vi "Separate_Bits.vi"(0 "JSON":string, 7 "int size number":u32, 11 "error in":errorcluster) -> (4 "Value_string":string, 8 "hex_data":string, 15 "error out":errorcluster)   [LabVIEW 2021]
uses:
  <vilib>/JDP Science/JSONtext/String Subset.vi
  <vilib>/JDP Science/JSONtext/support/Strip Quotes and Unescape.vi
  <vilib>/JDP Science/JSONtext/support/Unescape JSON string.vi
  <vilib>/JDP Science/JSONtext/Parsing/Parse Full Path or Item Name.vi
  <vilib>/JDP Science/JSONtext/Offset/Find Item Locations by Path.vi
  <vilib>/JDP Science/JSONtext/JSONtext.lvlib
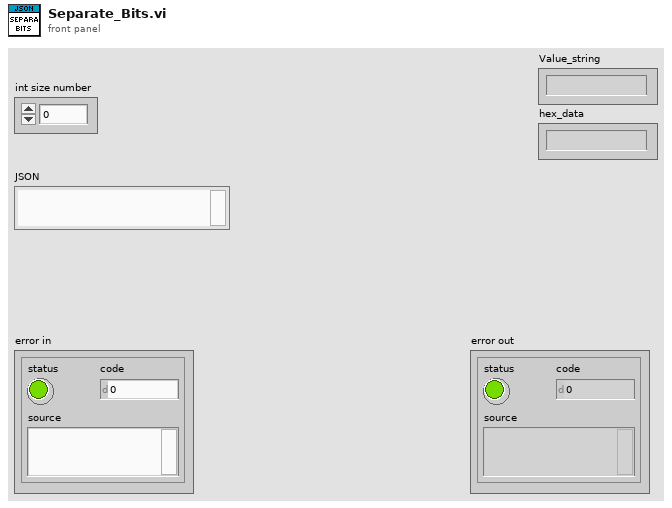
[diagram p1: front panel]
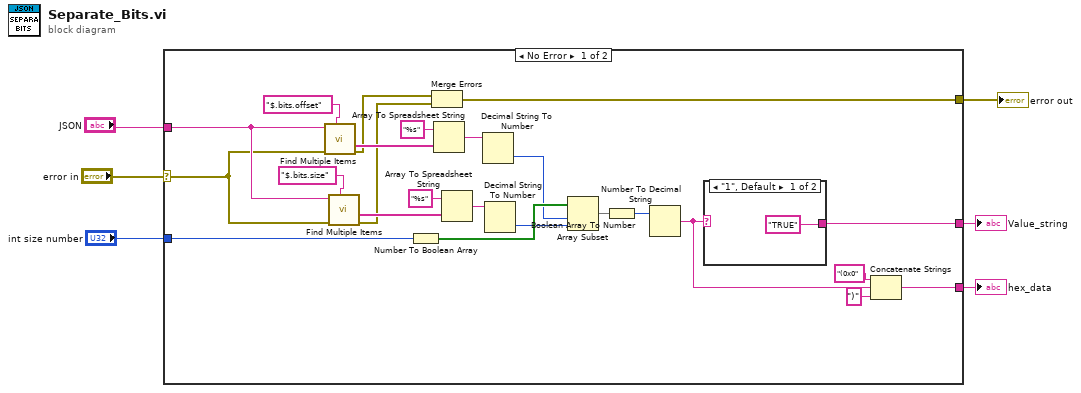
[diagram p0: block diagram]
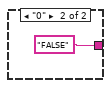
[diagram p2: hidden frame]
diagram:
  n1 = case shown="No Error" "error in" {
    selector: "error in" -> [w13 w33]
    tunnel: "int size number" -> [w15 _]
    tunnel: "JSON" -> [w14 _]
    tunnel: [w12 _] -> w2
    tunnel: [w11 _] -> w1
    tunnel: [w8 w33] -> w3
    frame No Error {
      n2 = call <vilib>:"Find Multiple Items.vi"("$Path or Item Name"="$.bits.offset", "error in (no error)"=w13, "JSON"=w14) -> ("error out"=w10:errorcluster, "<JSON>"=w19:string[])  [unwired: 5 in, 2 out]
      n3 = call <vilib>:"Find Multiple Items.vi"("$Path or Item Name"="$.bits.size", "error in (no error)"=w13, "JSON"=w14) -> ("error out"=w9:errorcluster, "<JSON>"=w24:string[])  [unwired: 5 in, 2 out]
      n4 = Number To Boolean Array(number=w15) -> (Boolean array=w28:bool[])
      n5 = Merge Errors(w10, w9) -> (w8:errorcluster)
      n6 = Array To Spreadsheet String(array=w19, 3:"%s" ("format string")) -> (spreadsheet string=w23:string)  [unwired: 1 in]
      n7 = Array To Spreadsheet String(array=w24, 3:"%s" ("format string")) -> (spreadsheet string=w22:string)  [unwired: 1 in]
      n8 = Decimal String To Number(string=w23) -> (number=w21:i32)  [unwired: 2 in, 1 out]
      n9 = Decimal String To Number(string=w22) -> (number=w20:i32)  [unwired: 2 in, 1 out]
      n10 = Array Subset(array=w28, index=w21, length=w20) -> (w30:bool[])
      n11 = Boolean Array To Number(Boolean array=w30) -> (number=w29:u32)
      n12 = Number To Decimal String(number=w29) -> (decimal integer string=w16:string)  [unwired: 1 in]
      n13 = case shown="\"1\", Default" w16 {
        tunnel: ["TRUE" "FALSE"] -> w12
        frame "1", Default {
        }
        frame "0" {
        }
      }
      n14 = Concatenate Strings("(0x0" ("string"), w16, ")" ("string")) -> (w11:string)
    }
    frame Error {
    }
  }
  "error out" <- w3
  "Value_string" <- w2
  "hex_data" <- w1
